vi "Initialize From Settings.vi"(8 "error in (no error)":errorcluster, 10 "settings":cluster{"key":string, "value":string}[](array[cluster]), 11 "Transfer Configuration in":refnum<class "Transfer Configuration.lvclass">) -> (0 "error out":errorcluster, 3 "Transfer Configuration out":refnum<class "Transfer Configuration.lvclass">)   [LabVIEW 2017, in "GE Reflective Memory.lvlib" / "Transfer Configuration.lvclass"]
uses:
  Transfer Configuration.lvclass
  Transfer Configuration.lvclass/Transfer Configuration.ctl
  GE Reflective Memory.lvlib
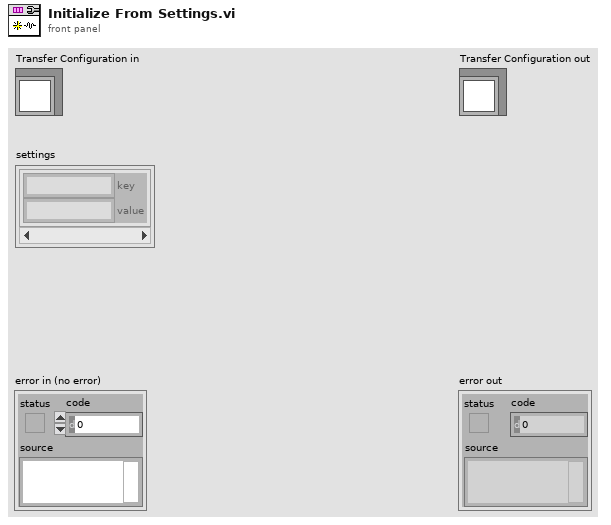
[diagram p1: front panel]
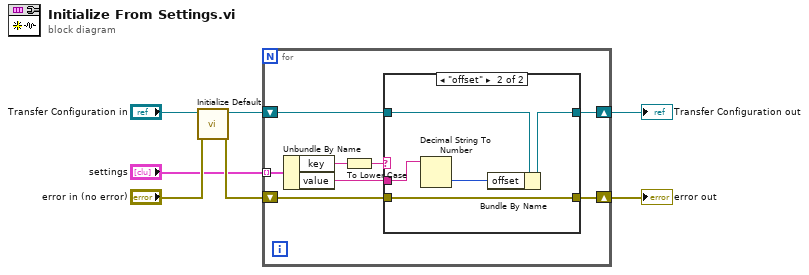
[diagram p0: block diagram]
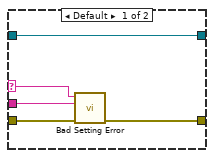
[diagram p2: hidden frame]
diagram:
  n1 = call-dynamic "Initialize Default.vi"("error in (no error)"="error in (no error)", "Transfer Configuration in"="Transfer Configuration in") -> ("error out"=w2:errorcluster, "Transfer Configuration out"=w4:refnum<class "Transfer Configuration.lvclass">)  [unwired: 8 in]
  n2 = for {
    shift-right: [w9] -> w6
    shift-left: w2 -> [w10]
    tunnel: "settings" -> [w15] mode=indexing
    shift-right: [w11] -> w7
    shift-left: w4 -> [w12]
    n3 = Unbundle By Name(w15) -> ("key"=w14:string, "value"=w8:string)
    n4 = To Lower Case(string=w14) -> (all lower case string=w13:string)
    n5 = case shown="\"offset\"" w13 {
      selector: w13 -> [w17 _]
      tunnel: w8 -> [w16 w22]
      tunnel: w12 -> [w18 w25]
      tunnel: [w18 w24] -> w11
      tunnel: w10 -> [w20 w23]
      tunnel: [w19 w23] -> w9
      frame Default {
        n6 = call "Bad Setting Error.vi"("error in (no error)"=w20, "value"=w16, "key"=w17) -> ("error out"=w19:errorcluster)  [unwired: 8 in]
      }
      frame "offset" {
        n7 = Decimal String To Number(string=w22) -> (number=w21:i32)  [unwired: 2 in, 1 out]
        n8 = Bundle By Name(cluster=w25, "offset"=w21) -> (w24:refnum<class "Transfer Configuration.lvclass">)
      }
    }
  }
  "error out" <- w6
  "Transfer Configuration out" <- w7
